vi "IndicatorChange.vi"() -> ()   [LabVIEW 2016]
uses:
  Controls/Boiler Status Indicators.ctl
panel:
  in  "Boiler Status Indicators":T1 {"Time Count" format="%.2g"}
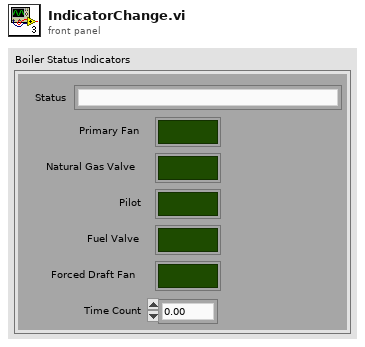
[diagram p1: front panel]
types:
  T1 = typedef "Boiler Status Indicators.ctl" = cluster{"Status":string, "Primary Fan":bool, "Natural Gas Valve":bool, "Pilot":bool, "Fuel Valve":bool, "Forced Draft Fan":bool, "Time Count":dbl}
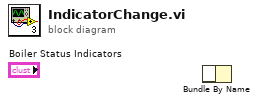
[diagram p0: block diagram]
diagram:
  n1 = Bundle By Name() -> ()  [unwired: 2 in, 1 out]
